vi "Get Controls from Tab Recursively.vi"(0 "PageSel Refnum":refnum<vi>, 11 "error in (no error)":errorcluster) -> (4 "Indicators in Tab":refnum<vi>[](array[refnum]), 6 "Controls in Tab":refnum<vi>[](array[refnum]), 15 "error out":errorcluster)   [LabVIEW 2021, in "Migrator.lvlib"]
uses:
  Migrator.lvlib
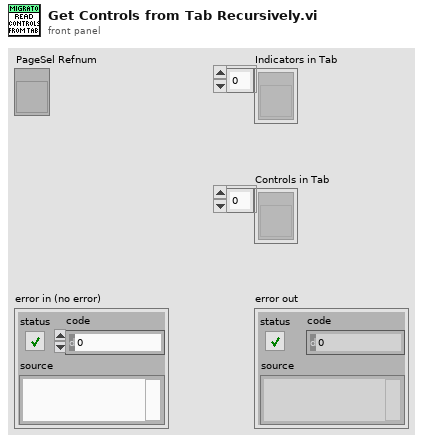
[diagram p1: front panel]
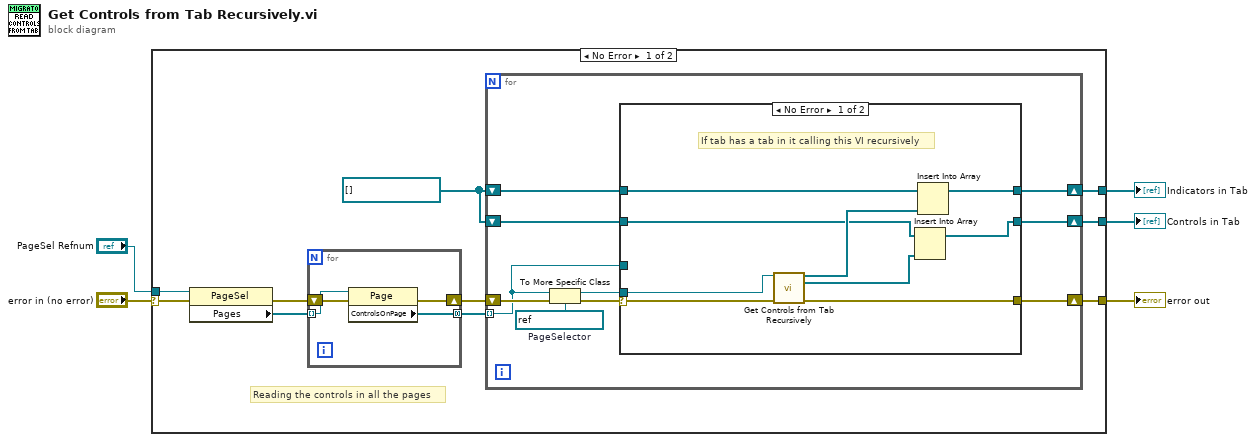
[diagram p0: block diagram]
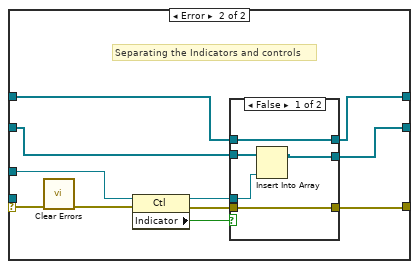
[diagram p2: hidden frame]
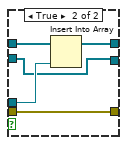
[diagram p3: hidden frame]
diagram:
  n1 = case shown="No Error" "error in (no error)" {
    selector: "error in (no error)" -> [w13 w60]
    tunnel: "PageSel Refnum" -> [w15 _]
    tunnel: [w10 _] -> w3
    tunnel: [w9 w60] -> w2
    tunnel: [w7 _] -> w1
    frame No Error {
      w6 = refnum<vi>[] []
      # "Reading the controls in all the pages"
      n2 = property class="PageSel"(reference=w15, error in=w13) -> (error out=w12:errorcluster, "Pages"=w14:refnum<vi>[])  [unwired: 1 out]
      n3 = for {
        tunnel: w14 -> [w19] mode=indexing
        tunnel: [w17] -> w8 mode=concatenating
        shift-right: [w16] -> w11
        shift-left: w12 -> [w18]
        n4 = property class="Page"(reference=w19, error in=w18) -> (error out=w16:errorcluster, "ControlsOnPage"=w17:refnum<vi>[])  [unwired: 1 out]
      }
      n5 = for {
        tunnel: w8 -> [w23] mode=indexing
        shift-right: [w24] -> w10
        shift-left: w6 -> [w26]
        shift-right: [w22] -> w9
        shift-left: w11 -> [w29]
        shift-right: [w20] -> w7
        shift-left: w6 -> [w21]
        w28 = refnum<vi> refnum  # PageSelector
        n6 = To More Specific Class(target class=w28, reference=w23, error in=w29) -> (specific class reference=w25:refnum<vi>, error out=w27:errorcluster)
        n7 = case shown="No Error" w27 {
          selector: w27 -> [w38 w49]
          tunnel: w26 -> [w35 w46]
          tunnel: w25 -> [w37 _]
          tunnel: [w34 w42] -> w24
          tunnel: w23 -> [_ w45]
          tunnel: [w36 w40] -> w22
          tunnel: w21 -> [w32 w43]
          tunnel: [w30 w41] -> w20
          frame No Error {
            # "If tab has a tab in it calling this VI recursively"
            n8 = call "Get Controls from Tab Recursively.vi"("PageSel Refnum"=w37, "error in (no error)"=w38) -> ("Indicators in Tab"=w33:refnum<vi>[], "Controls in Tab"=w31:refnum<vi>[], "error out"=w36:errorcluster)  [unwired: 11 in]
            n9 = Insert Into Array(array=w32, new element=w31) -> (w30:refnum<vi>[])  [unwired: 1 in]
            n10 = Insert Into Array(array=w35, new element=w33) -> (w34:refnum<vi>[])  [unwired: 1 in]
          }
          frame Error {
            # "Separating the Indicators and controls"
            n11 = call <vilib>:"Clear Errors.vi"("error in (no error)"=w49) -> ("error out"=w48:errorcluster)  [unwired: 5 in, 1 out]
            n12 = property class="Ctl"(reference=w45, error in=w48) -> (reference out=w44:refnum<vi>, error out=w39:errorcluster, "Indicator"=w47:bool)
            n13 = case shown="False" w47 {
              tunnel: w46 -> [w54 w59]
              tunnel: [w54 w58] -> w42
              tunnel: w44 -> [w52 w57]
              tunnel: w43 -> [w53 w56]
              tunnel: [w51 w56] -> w41
              tunnel: [w50 w55] -> w40
              tunnel: w39 -> [w50 w55]
              frame False {
                n14 = Insert Into Array(array=w53, new element=w52) -> (w51:refnum<vi>[])  [unwired: 1 in]
              }
              frame True {
                n15 = Insert Into Array(array=w59, new element=w57) -> (w58:refnum<vi>[])  [unwired: 1 in]
              }
            }
          }
        }
      }
    }
    frame Error {
    }
  }
  "error out" <- w2
  "Indicators in Tab" <- w3
  "Controls in Tab" <- w1
